vi "Abort.vi"(8 "Error In":errorcluster, 11 "AutoData":T1) -> (0 "Error Out":errorcluster, 3 "AutoData out":T1)   [LabVIEW 2019, in "AutoMode.lvlib"]
uses:
  AutoMode.lvlib
  Cluster - AutoModeData.ctl
  MainController/Cluster - TestSettings.ctl
  MainController/Cluster - HardwareConfiguration.ctl
  MainController/Cluster - TestResults.ctl
  Cluster - AutoModeMessage.ctl
  Enum - AutoModeState.ctl
  MainController/Cluster - MainControllerMessage.ctl
  MainController/Enum - MainState.ctl
  Mark10 API/WriteStopMove.vi
  MainController/MainController.lvlib
  Mark10 API/Mark 10 TSTM-DC.lvlib
  EventLogger/EventLogger.lvlib
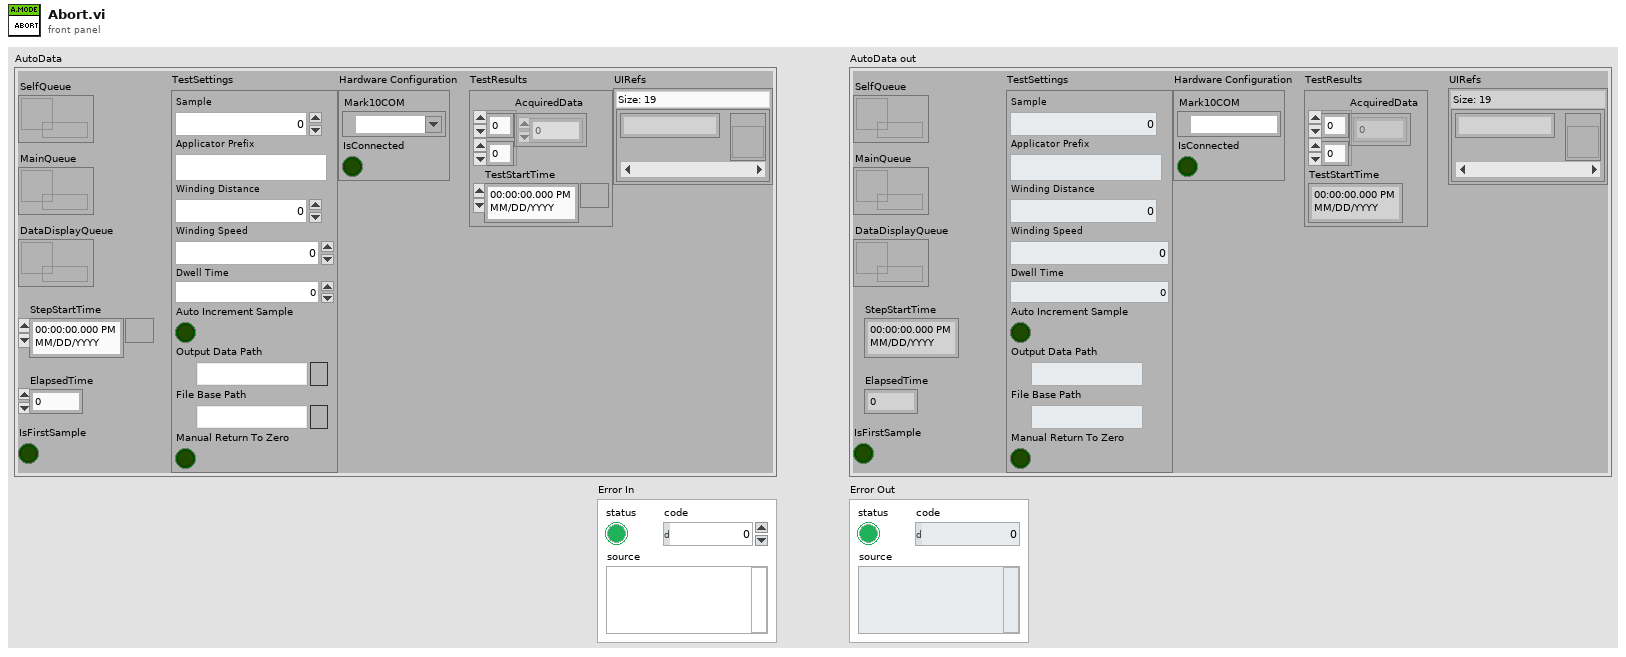
[diagram p1: front panel]
types:
  T1 = typedef "AutoMode.lvlib/Cluster - AutoModeData.ctl" = cluster{"DataDisplayQueue":refnum<queue>, "StepStartTime":timestamp, "TestSettings":T2, "Hardware Configuration":T3, "TestResults":T4, "ElapsedTime":dbl, "IsFirstSample":bool, "UIRefs":map{string, refnum<vi>}, "SelfQueue":refnum<queue>, "MainQueue":refnum<queue>}
  T2 = typedef "MainController.lvlib/Cluster - TestSettings.ctl" = cluster{"Sample":u32, "Applicator Prefix":string, "Winding Distance":dbl, "Winding Speed":dbl, "Dwell Time":dbl, "Auto Increment Sample":bool, "Output Data Path":path, "File Base Path":path, "Manual Return To Zero":bool}
  T3 = typedef "MainController.lvlib/Cluster - HardwareConfiguration.ctl" = cluster{"Mark10COM":refnum<visa-resource-name>, "IsConnected":bool}
  T4 = typedef "MainController.lvlib/Cluster - TestResults.ctl" = cluster{"AcquiredData":dbl[][], "TestStartTime":timestamp}
  T5 = typedef "MainController.lvlib/Enum - MainState.ctl" = enum16{"Initialize", "InitUIRefs", "LaunchSettings", "LaunchAutoMode", "LaunchManualMode", "LaunchTestReport", "ConnectHardware", "DisconnectHardware", "HiliteNavItems", "StartAutoMode", "PauseAutoMode", "StopAutoMode", "ShowFlyout", "HideFlyout", "BroadcastSettings", "PickupTestSettings", "BroadcastHW", "AutoTestDone", "DAQStatus", "UpdateCommandBar", "Error", "RecieveError", "Exit"}
  T6 = typedef "AutoMode.lvlib/Enum - AutoModeState.ctl" = enum16{"Initialize", "Idle", "UpdateConfig", "UpdateHWConfig", "BroadcastSettings", "Start", "CheckValidReportPath", "Winding", "WaitForWinding", "Unwind", "WaitForUnwind", "Stop", "Abort", "WriteDataToFile", "EventTriggered", "GenerateFilePath", "ZeroPosition", "GotoZero", "Error", "Exit"}
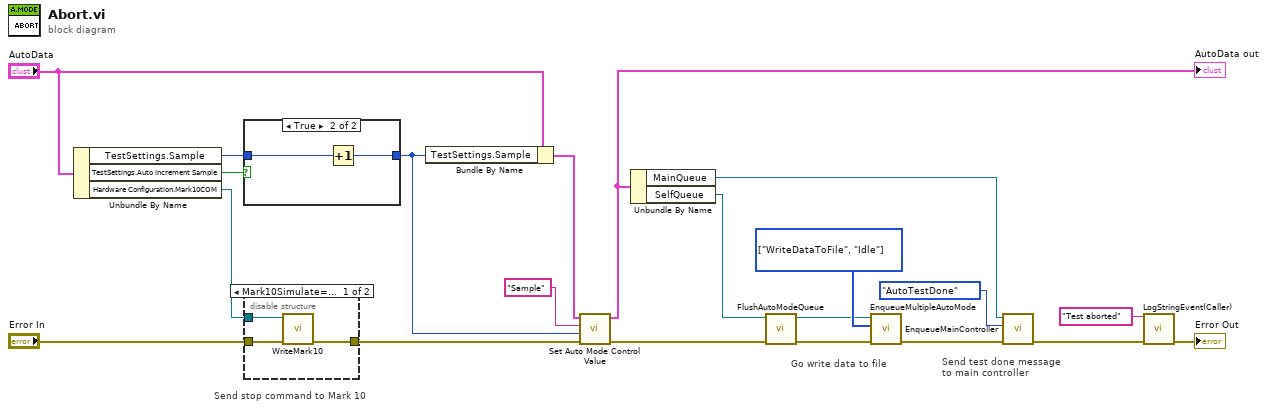
[diagram p0: block diagram]
diagram:
  w19 = T6[] [enum."WriteDataToFile", enum."Idle"] items=["Initialize", "Idle", "UpdateConfig", "UpdateHWConfig", "BroadcastSettings", "Start", "CheckValidReportPath", "Winding", "WaitForWinding", "Unwind", "WaitForUnwind", "Stop", "Abort", "WriteDataToFile", "EventTriggered", "GenerateFilePath", "ZeroPosition", "GotoZero", "Error", "Exit"] ("CycleTestState")
  # "Send test done message to main controller"
  # "Go write data to file"
  # "Send stop command to Mark 10"
  n1 = Unbundle By Name("AutoData") -> ("TestSettings.Sample"=w15:u32, "TestSettings.Auto Increment Sample"=w16:bool, "Hardware Configuration.Mark10COM"=w20:refnum<visa-resource-name>)
  n2 = case shown="True" w16 {
    tunnel: w15 -> [w22 w24]
    tunnel: [w22 w23] -> w6
    frame False {
    }
    frame True {
      n3 = Increment(x=w24) -> (x+1=w23:u32)
    }
  }
  n4 = disable-structure shown="Mark10Simulate==False, Default" {
    disable-tunnel: "Error In" -> [w27 w28]
    disable-tunnel: [w26 w28] -> w21
    disable-tunnel: w20 -> [w25 _]
    frame condition #0 (active) {
      n5 = call-poly "WriteMark10.vi"("error in"=w27, "VISA resource name"=w25) -> ("error out"=w26:errorcluster)  [unwired: 8 in, 1 out]
    }
    frame condition #1 {
    }
  }
  n6 = Bundle By Name(cluster="AutoData", "TestSettings.Sample"=w6) -> (w9:T1)
  n7 = call "Set Auto Mode Control Value.vi"("Error In"=w21, "Value"=w6, "key"="Sample", "AutoData"=w9) -> ("Error Out"=w10:errorcluster, "AutoData out"=w8:T1)  [unwired: 6 in]
  "AutoData out" <- w8
  n8 = Unbundle By Name(w8) -> ("MainQueue"=w14:refnum<queue>, "SelfQueue"=w4:refnum<queue>)
  n9 = call "FlushAutoModeQueue.vi"("error in (no error)"=w10, "Queue in"=w4) -> ("error out"=w5:errorcluster, "Queue out"=w3:refnum<queue>)  [unwired: 8 in]
  n10 = call "EnqueueMultipleAutoMode.vi"("error in (no error)"=w5, "AutoState"=w19, "Queue in"=w3) -> ("error out"=w18:errorcluster)  [unwired: 7 in, 1 out]
  n11 = call "EnqueueMainController.vi"("error in (no error)"=w18, "Message"=Enum_-_MainState."AutoTestDone", "MainQueue"=w14) -> ("error out"=w12:errorcluster)  [unwired: 6 in, 2 out]
  n12 = call "LogStringEvent(Caller).vi"("Error In"=w12, "Field"="Test aborted") -> ("Error Out"=→"Error Out":errorcluster)  [unwired: 9 in]
